vi "Yokogawa WT1800 Series Acquire Multiple Waveform.vi"() -> ()   [LabVIEW 2015]
doc: "This example shows how to configure multiple traces and acquire waveforms from multiple traces."
uses:
  <instrlib>/Yokogawa WT1800 Series/Public/Configure/Configure Range (Voltage).vi
  <instrlib>/Yokogawa WT1800 Series/Public/Configure/Configure Range (Current 50A).vi
  <instrlib>/Yokogawa WT1800 Series/Public/Data/Read Waveform (Multiple).vi
  <instrlib>/Yokogawa WT1800 Series/Yokogawa WT1800 Series.lvlib
panel:
  in  "Trace (0: U1)":i32[](array[ring]) items=["U1", "I1", "U2", "I2", "U3", "I3", "U4", "I4", "U5", "I5", "U6", "I6", "Speed", "Torque", "AUX1", "AUX2"]
  in  "Element (0: ALL)":i32(ring) items=["All", "1", "2", "3", "4", "5", "6"]
  in  "Current 50A Range (50A <25A>)":dbl(ring)=25.0 items=["1 <500m>"=0.5, "2 <1>"=1.0, "5 <2.5>"=2.5, "10 <5>"=5.0, "20 <10>"=10.0, "50 <25>"=25.0]
  in  "Voltage Range (1000V <500V>)":dbl(ring)=500.0 items=["1.5 <7.5>"=0.75, "3 <1.5>"=1.5, "6 <3>"=3.0, "10 <5>"=5.0, "15 <7.5>"=7.5, "30 <15>"=15.0, "60 <30>"=30.0, "100 <50>"=50.0, "150 <75>"=75.0, "300 <150>"=150.0, "600 <300>"=300.0, "1000 <500>"=500.0]
  in  "Timeout (10000 ms)":i32=10000 min=1
  in  "VISA resource name":refnum<visa-resource-name>
  out "Waveform Graph":T1(graph)
  # "(c) 2011 Yokogawa Meters & Instruments Corporation.  All rights reserved."
  # "WT1800 SERIES POWER ANALYZER"
  # "ms"
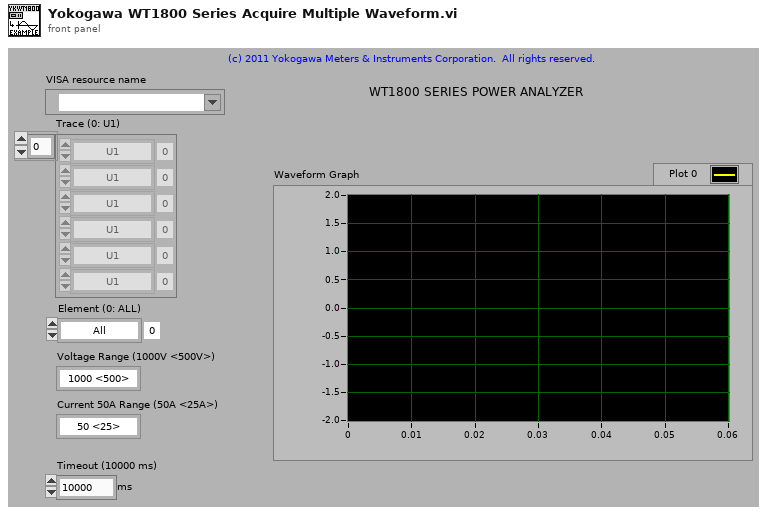
[diagram p1: front panel]
types:
  T1 = cluster{"start":dbl, "Sampling Time":dbl, "Output":dbl[]}[]
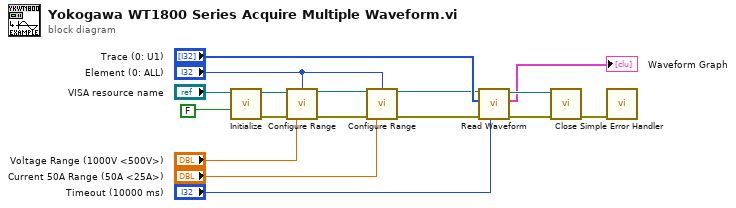
[diagram p0: block diagram]
diagram:
  n1 = call <instrlib>:"Initialize.vi"("Reset (True)"=FALSE, "VISA resource name"="VISA resource name") -> ("error out"=w4:errorcluster, "VISA resource name out"=w5:refnum<visa-resource-name>)  [unwired: 8 in]
  n2 = call-poly <instrlib>:"Configure Range.vi"("VISA resource name"=w5, "Element (0:All)"="Element (0: ALL)", "error in (no error)"=w4, "Manual Range (1000 <500> V)"="Voltage Range (1000V <500V>)") -> ("VISA resource name out"=w15:refnum<visa-resource-name>, "error out"=w14:errorcluster)  [unwired: 10 in]
  n3 = call-poly <instrlib>:"Configure Range.vi"("VISA resource name"=w15, "Element (0:All)"="Element (0: ALL)", "error in (no error)"=w14, "Manual Range (50 <25> A)"="Current 50A Range (50A <25A>)") -> ("VISA resource name out"=w7:refnum<visa-resource-name>, "error out"=w6:errorcluster)  [unwired: 10 in]
  n4 = call-poly <instrlib>:"Read Waveform.vi"("Timeout (10000 ms)"="Timeout (10000 ms)", "error in (no error)"=w6, "Trace (0: U1)"="Trace (0: U1)", "VISA resource name"=w7) -> ("error out"=w12:errorcluster, "Waveform Data"=→"Waveform Graph":T1, "VISA resource name out"=w13:refnum<visa-resource-name>)  [unwired: 5 in]
  n5 = call <instrlib>:"Close.vi"("error in (no error)"=w12, "VISA resource name"=w13) -> ("error out"=w11:errorcluster)  [unwired: 9 in]
  n6 = call <vilib>:"Simple Error Handler.vi"("error in (no error)"=w11) -> ()  [unwired: 4 in, 5 out]
